vi "stateC.vi"(3 "Stop/Transfer":bool, 4 "State":enum16{"Stopped", "Foward", "Reverse"}(ring), 5 "Start":bool) -> (0 "Ball State":enum16{"Occupied", "Vacant"}(ring), 1 "OutState":enum16{"Stopped", "Foward", "Reverse"}(ring))   [LabVIEW 2011]
panel:
  in  "Ball state":enum16{"Occupied", "Vacant"}(ring)
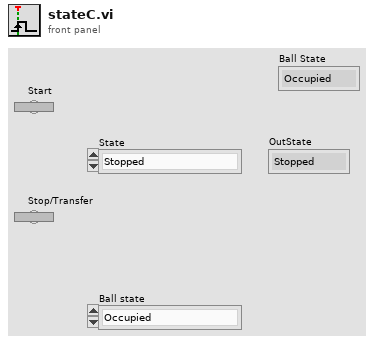
[diagram p1: front panel]
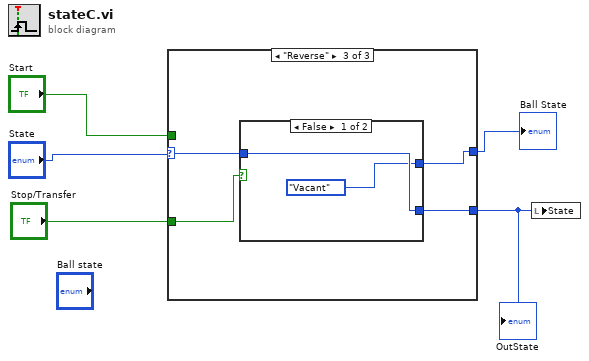
[diagram p0: block diagram]
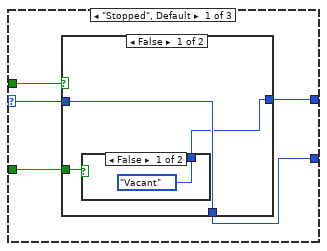
[diagram p2: hidden frame]
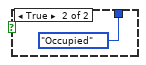
[diagram p3: hidden frame]
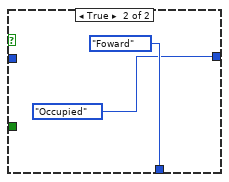
[diagram p4: hidden frame]
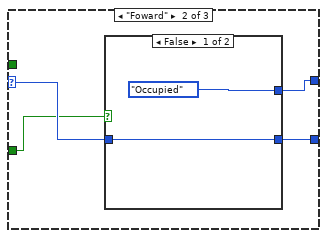
[diagram p5: hidden frame]
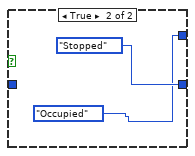
[diagram p6: hidden frame]
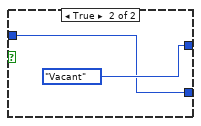
[diagram p7: hidden frame]
diagram:
  n1 = case shown="\"Reverse\"" "State" {
    selector: "State" -> [w8 w20 w27]
    tunnel: "Start" -> [w10 _ _]
    tunnel: [w9 w21 w28] -> w4
    tunnel: "Stop/Transfer" -> [w6 w19 w29]
    tunnel: [w7 w18 w26] -> w1
    frame "Stopped", Default {
      n2 = case shown="False" w10 {
        tunnel: [w13 enum16{"Stopped", "Foward"}."Foward" ("State")] -> w9
        tunnel: w8 -> [w13 _]
        tunnel: [w12 enum16{"Occupied", "Vacant"}."Occupied" ("State")] -> w7
        tunnel: w6 -> [w11 _]
        frame False {
          n3 = case shown="False" w11 {
            tunnel: [enum16{"Occupied", "Vacant"}."Vacant" ("State") enum16{"Occupied", "Vacant"}."Occupied" ("State")] -> w12
            frame False {
            }
            frame True {
            }
          }
        }
        frame True {
        }
      }
    }
    frame "Foward" {
      n4 = case shown="False" w19 {
        tunnel: [w23 enum16{"Stopped", "Running"}."Stopped" ("x")] -> w21
        tunnel: w20 -> [w23 _]
        tunnel: [enum16{"Occupied", "Vacant"}."Occupied" ("State") enum16{"Occupied", "Vacant"}."Occupied" ("State")] -> w18
        frame False {
        }
        frame True {
        }
      }
    }
    frame "Reverse" {
      n5 = case shown="False" w29 {
        tunnel: [w31 w32] -> w28
        tunnel: w27 -> [w31 w32]
        tunnel: [enum16{"Occupied", "Vacant"}."Vacant" ("State") enum16{"Occupied", "Vacant"}."Vacant" ("State")] -> w26
        frame False {
        }
        frame True {
        }
      }
    }
  }
  "OutState" <- w4
  "Ball State" <- w1
  n6 = local write "State"(w4) -> ()
